vi "Advance.vi"(8 "error in (no error)":errorcluster, 11 "PathTokenizer in":refnum<class "PathTokenizer.lvclass">) -> (0 "error out":errorcluster, 3 "PathTokenizer out":refnum<class "PathTokenizer.lvclass">)   [LabVIEW 2019, in "PathTokenizer.lvclass"]
uses:
  PathTokenizer.lvclass
  PathTokenizer.lvclass/PathTokenizer.ctl
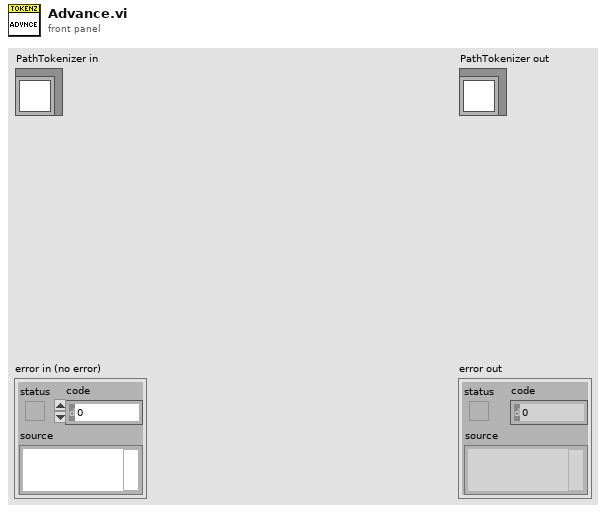
[diagram p1: front panel]
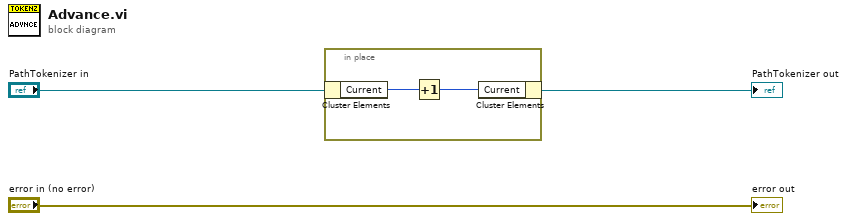
[diagram p0: block diagram]
diagram:
  n1 = in-place "In Place Element Structure" {
    n2 = in-place-cluster #1("PathTokenizer in") -> ("Current"=w5:i32)
    n3 = Increment(x=w5) -> (x+1=w4:i32)
    n4 = in-place-cluster #1("Current"=w4) -> (→"PathTokenizer out":refnum<class "PathTokenizer.lvclass">)
  }
  "error out" <- "error in (no error)"
